vi "ziExample-ReadSingleValue.vi"(0 "Address":string="DEV", 1 "oscs/*/freq":dbl=12345.0 caption="Frequency (Hz)" format="%#_6p", 2 "demods/0/timeconstant":dbl=0.001 caption="TC (s)" format="%#_6p", 3 "phaseshift":dbl=12.0 caption="Phase (deg)" format="%#_6p", 4 "demods/0/harmonic":dbl caption="Harmonic", 5 "Load Settings Path":string, 6 "Save Settings Path":string, 7 "Load":bool, 8 "Save":bool, 10 "stop":bool) -> (20 "Time since last boot (s)":dbl, 21 "R (Vrms)":dbl format="%#_4g", 22 "Theta (rad)":dbl, 23 "Demod Sample Out":T1, 24 "Selected Device":string)   [LabVIEW 2009]
doc: "Control a Zurich instrument device via the LabOne Labview API. \nRequirements: Zurich Instruments MFLI, HF2 or UHFLI \nExample from the Getting Started guide: A single demodulator value is read and unbundled read timestamp, X and Y.\n\n© Zurich Instruments AG, www.zhinst.com"
uses:
  <instrlib>/Zurich Instruments LabOne/Public/Configure/ziSetValueDoubleArray.vi
  <instrlib>/Zurich Instruments LabOne/Public/Utility/ziTicksToS_single.vi
  <instrlib>/Zurich Instruments LabOne/Zurich Instruments LabOne.lvlib
panel:
  out "Error Out":errorcluster
  # "This example describes how ziGetValueDemodSample.vi can be used"
  # "GetValueDemodSample output"
  # "ziExample-ReadSingleValue.vi\nRequirements: HF2, UHFLI or MFLI\nsee block diagram for VI description"
  # "Settings"
  # "Unbundled output"
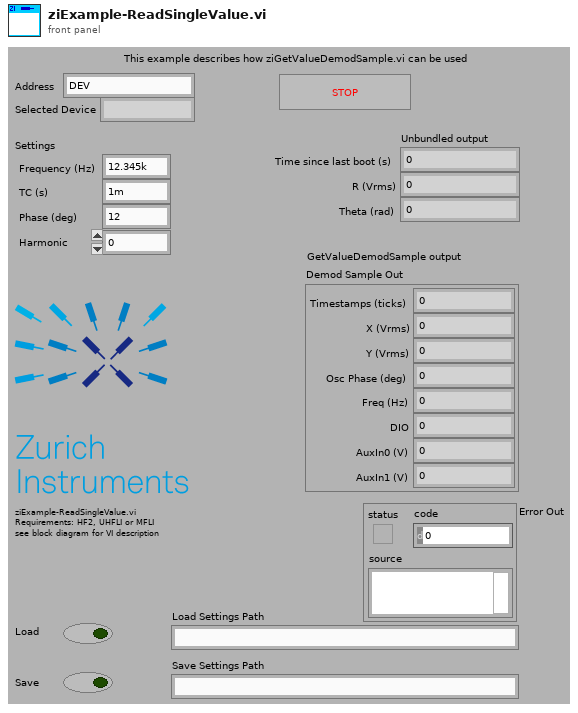
[diagram p1: front panel]
types:
  T1 = cluster{"Timestamps (ticks)":u64, "X (Vrms)":dbl, "Y (Vrms)":dbl, "Osc Phase (deg)":dbl, "Freq (Hz)":dbl, "DIO":u32, "AuxIn0 (V)":dbl, "AuxIn1 (V)":dbl}
  T2 = typedef "Zurich Instruments LabOne.lvlib/ziTypeHandle.ctl" = cluster{"handleValid":bool, "Conn":u64, "Path Prefix":string, "Handle":u64, "Connected":bool, "Clockbase(s)":dbl}
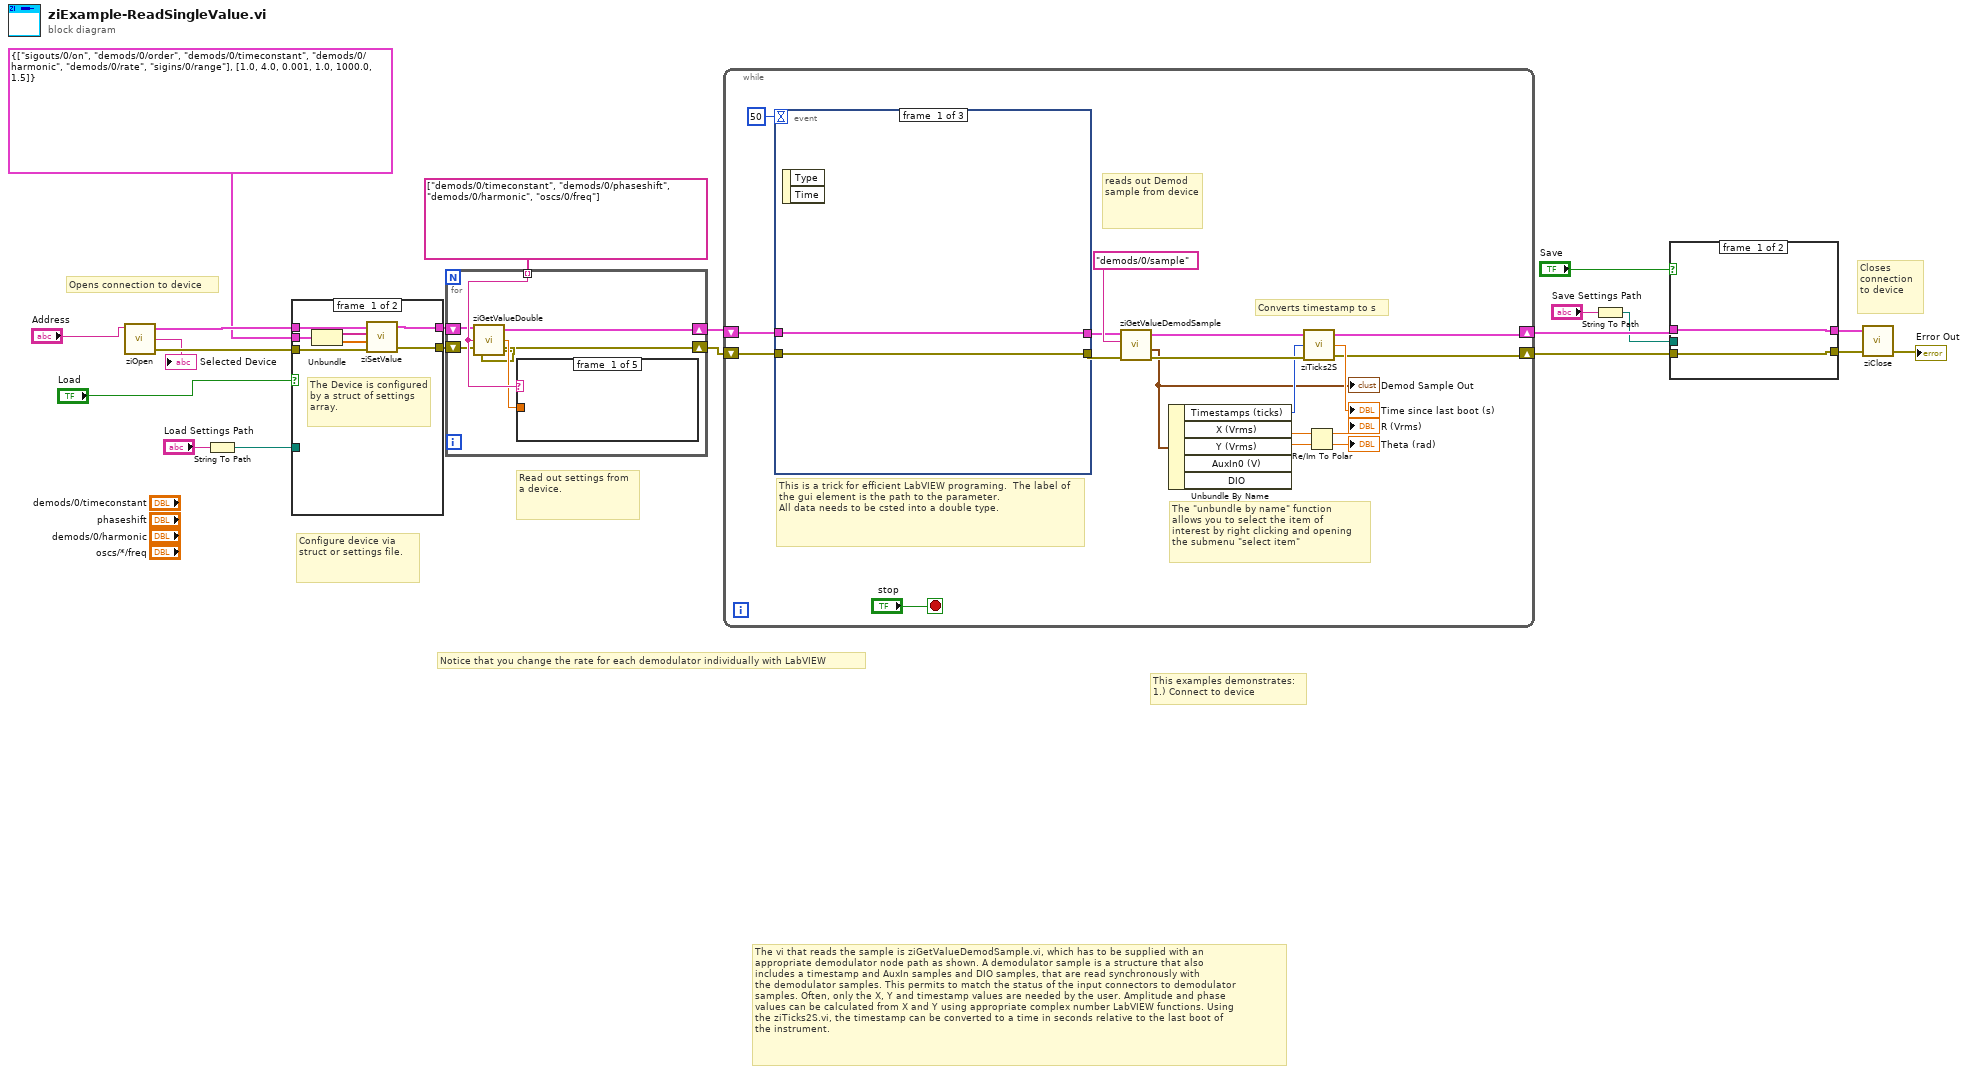
[diagram p0: block diagram]
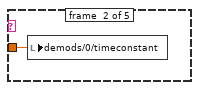
[diagram p2: hidden frame]
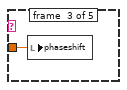
[diagram p3: hidden frame]
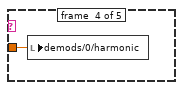
[diagram p4: hidden frame]
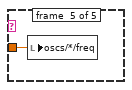
[diagram p5: hidden frame]
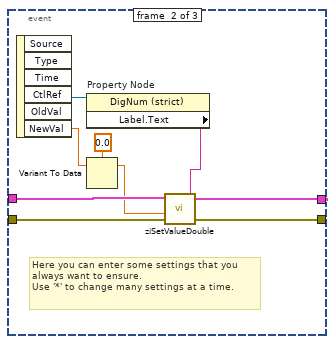
[diagram p6: hidden frame]
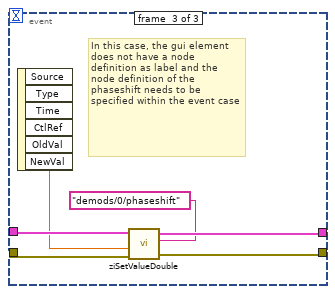
[diagram p7: hidden frame]
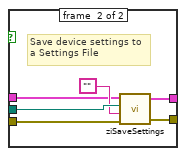
[diagram p8: hidden frame]
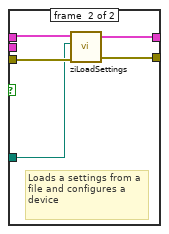
[diagram p9: hidden frame]
diagram:
  # "Closes connection to device"
  # "Opens connection to device"
  # "Read out settings from a device."
  # "Configure device via struct or settings file."
  # "This examples demonstrates:\n1.) Connect to device"
  # "Notice that you change the rate for each demodulator individually with LabVIEW"
  # "The vi that reads the sample is ziGetValueDemodSample.vi, which has to be supplied with an \nappropriate demodulator node path as shown. A demodulator sample is a structure that also \nincludes a timestamp and AuxIn samples and DIO samples, that are read synchronously with \nthe demodulator samples. This permits to match the status of the input connectors to demodulator \nsamples. Often, only the X, Y and timestamp values are needed by the user. Amplitude and phase\nvalues can be calculated from X and Y using appropriate complex number LabVIEW functions. Using \nthe ziTicks2S.vi, the timestamp can be converted to a time in seconds relative to the last boot of \nthe instrument."
  n1 = call <instrlib>:"ziOpen.vi"("Address"="Address") -> ("Error Out"=w20:errorcluster, "Selected Device"=→"Selected Device":string, "HandleOut"=w21:T2)  [unwired: 3 in]
  n2 = String To Path(string="Load Settings Path") -> (path=w4:path)
  n3 = case shown="True" "Load" {
    tunnel: w20 -> [w28 w33]
    tunnel: w21 -> [w27 w30]
    tunnel: [w26 w31] -> w9
    tunnel: [w25 w32] -> w8
    tunnel: cluster{string[], dbl[]} {["sigouts/0/on", "demods/0/order", "demods/0/timeconstant", "demods/0/harmonic", "demods/0/rate", "sigins/0/range"], [1.0, 4.0, 0.001, 1.0, 1000.0, 1.5]} -> [w24 _]
    tunnel: w4 -> [_ w29]
    frame #0 {
      # "The Device is configured by a struct of settings array."
      n4 = Unbundle(w24) -> (w23:string[], w22:dbl[])
      n5 = call-poly <instrlib>:"ziSetValue.vi"("Error In"=w28, "Values"=w22, "Paths"=w23, "Handle In"=w27) -> ("Error Out"=w25:errorcluster, "Handle Out"=w26:T2)  [unwired: 1 in]
    }
    frame #1 {
      # "Loads a settings from a file and configures a device"
      n6 = call <instrlib>:"ziLoadSettings.vi"("Error in"=w33, "File path (dialog if empty)"=w29, "Handle in"=w30) -> ("Error out"=w32:errorcluster, "Handle out"=w31:T2)  [unwired: 2 in]
    }
  }
  n7 = for {
    tunnel: string[] ["demods/0/timeconstant", "demods/0/phaseshift", "demods/0/harmonic", "oscs/0/freq"] -> [w39] mode=indexing
    shift-right: [w35] -> w7
    shift-left: w9 -> [w37]
    shift-right: [w34] -> w6
    shift-left: w8 -> [w36]
    n8 = call <instrlib>:"ziGetValueDouble.vi"("error in"=w36, "Path"=w39, "Handle in"=w37) -> ("error out"=w34:errorcluster, "Value"=w38:dbl, "Handle out"=w35:T2)
    n9 = case shown="\"oscs/0/freq\"" w39 {
      tunnel: w38 -> [_ w40 w41 w42 w43]
      frame #0 {
      }
      frame #1 {
        n10 = local write "demods/0/timeconstant"(w40) -> ()
      }
      frame #2 {
        n11 = local write "phaseshift"(w41) -> ()
      }
      frame #3 {
        n12 = local write "demods/0/harmonic"(w42) -> ()
      }
      frame #4 {
        n13 = local write "oscs/*/freq"(w43) -> ()
      }
    }
  }
  n14 = while {
    shift-right: [w46] -> w13
    shift-left: w7 -> [w59]
    shift-right: [w45] -> w14
    shift-left: w6 -> [w61]
    stop <- "stop" stop-if-true
    # "Converts timestamp to s"
    # "reads out Demod sample from device"
    # "This is a trick for efficient LabVIEW programing.  The label of the gui element is the path to the parameter.\nAll data needs to be csted into a double type."
    # "The \"unbundle by name\" function\nallows you to select the item of \ninterest by right clicking and opening\nthe submenu \"select item\""
    n15 = event shown="[1] \"oscs/*/freq\", \"demods/0/harmonic\", \"demods/0/timeconstant\": Value Change" {
      selector: _ -> [_ _ _]
      dyn-events: _ -> [_ _ _]
      timeout: 50 -> [_ _ _]
      tunnel: w59 -> [w63 w70 w77]
      tunnel: w61 -> [w62 w67 w76]
      tunnel: [w63 w69 w78] -> w47
      tunnel: [w62 w68 w75] -> w48
      event #0 {
        n16 = event-data() -> ()  [unwired: 3 out]
      }
      event #1 {
        # "Here you can enter some settings that you always want to ensure.\nUse '*' to change many settings at a time."
        n17 = event-data() -> ("CtlRef"=w72:refnum<vi>, "NewVal"=w71:dbl)  [unwired: 5 out]
        n18 = property on="Property Node" class="DigNum (strict)"(reference=w72) -> ("Label.Text"=w64:string)  [unwired: 1 in, 2 out]
        n19 = Variant To Data(Variant=w71, type=0.0 ("demods/")) -> (data=w66:dbl)  [unwired: 1 in, 1 out]
        n20 = call <instrlib>:"ziSetValueDouble.vi"("Error In"=w67, "Value"=w66, "Path"=w64, "Handle In"=w70) -> ("Error Out"=w68:errorcluster, "Handle Out"=w69:T2)  [unwired: 1 out]
      }
      event #2 {
        # "In this case, the gui element does not have a node definition as label and the node definition of the phaseshift needs to be\nspecified within the event case"
        n21 = event-data() -> ("NewVal"=w73:dbl)  [unwired: 6 out]
        n22 = call <instrlib>:"ziSetValueDouble.vi"("Error In"=w76, "Value"=w73, "Path"="demods/0/phaseshift", "Handle In"=w77) -> ("Error Out"=w75:errorcluster, "Handle Out"=w78:T2)  [unwired: 1 out]
      }
    }
    n23 = call <instrlib>:"ziGetValueDemodSample.vi"("error in"=w48, "Path"="demods/0/sample", "Handle In"=w47) -> ("error out"=w58:errorcluster, "Demod Sample Out"=w53:T1, "Handle Out"=w57:T2)  [unwired: 2 in]
    "Demod Sample Out" <- w53
    n24 = Unbundle By Name(w53) -> ("Timestamps (ticks)"=w55:u64, "X (Vrms)"=w49:dbl, "Y (Vrms)"=w50:dbl)  [unwired: 2 out]
    n25 = call-poly <instrlib>:"ziTicks2S.vi"("Error In"=w58, "Timestamp(ticks)"=w55, "Handle In"=w57) -> ("Error Out"=w45:errorcluster, "Timestamp(s)"=→"Time since last boot (s)":dbl, "Handle Out"=w46:T2)
    n26 = Re/Im To Polar(2:w50, 3:w49) -> (0:→"Theta (rad)":dbl, 1:→"R (Vrms)":dbl)
  }
  n27 = String To Path(string="Save Settings Path") -> (path=w3:path)
  n28 = case shown="True" "Save" {
    tunnel: [w79 w85] -> w17
    tunnel: [w80 w84] -> w16
    tunnel: w3 -> [_ w86]
    tunnel: w14 -> [w80 w82]
    tunnel: w13 -> [w79 w81]
    frame #0 {
    }
    frame #1 {
      # "Save device settings to\na Settings File"
      n29 = call <instrlib>:"ziSaveSettings.vi"("Error In"=w82, "Path (\"\")"="", "file path (dialog if empty)"=w86, "Handle In"=w81) -> ("Error Out"=w84:errorcluster, "Handle Out"=w85:T2)  [unwired: 1 out]
    }
  }
  n30 = call <instrlib>:"ziClose.vi"("Error In"=w16, "Handle In"=w17) -> ("Error Out"=→"Error Out":errorcluster)  [unwired: 2 in, 1 out]
